vi "Galil_addresses.vi"() -> ()   [LabVIEW 2011]
panel:
  in  "Galil.IGalil":refnum<k7>
  out "addresses":string[](array[string])
  out "Library Version:":string
  out "error out":errorcluster
  # "This vi Shows how to use the addresses member of the Galil Communications Library.  \n\nThis will list all of the available controllers on the PC/network"
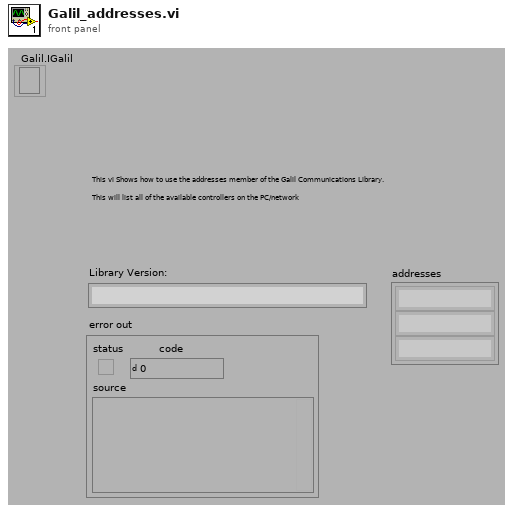
[diagram p1: front panel]
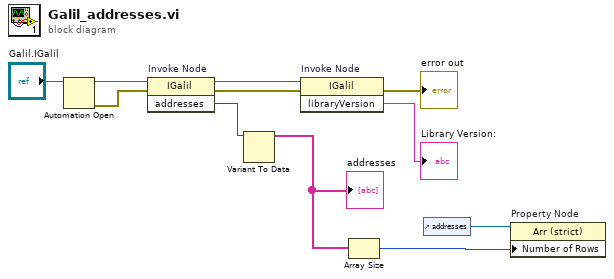
[diagram p0: block diagram]
diagram:
  n1 = Automation Open(Automation Refnum="Galil.IGalil") -> (Automation Refnum=w9:refnum<k7>, error out=w8:errorcluster)  [unwired: 1 in, 2 out]
  n2 = invoke on="Invoke Node" class="IGalil" method="addresses"(reference=w9, error in=w8) -> (reference out=w11:refnum<k7>, error out=w7:errorcluster, "addresses"=w6:variant)  [unwired: 1 in]
  n3 = Variant To Data(Variant=w6) -> (data=w4:string[])  [unwired: 2 in, 1 out]
  "addresses" <- w4
  n4 = invoke on="Invoke Node" class="IGalil" method="libraryVersion"(reference=w11, error in=w7) -> (error out=→"error out":errorcluster, "libraryVersion"=→"Library Version:":string)  [unwired: 1 in, 1 out]
  n5 = Array Size(array=w4) -> (size(s)=w2:i32)
  n6 = control-ref of="addresses"() -> (w3:refnum<vi>)
  n7 = property on="Property Node" class="Arr (strict)"(reference=w3, "Number of Rows"=w2) -> ()  [unwired: 1 in, 2 out]
